vi "16_LinesDecoder.vi"(3 "ENABLED":bool=TRUE, 4 "Integer 0..15  (0)":i32 min=0 max=15) -> (1 "decoded drives":T1)   [LabVIEW 2012]
doc: "Used by Scanner with R and T displays.vi."
panel:
  # "Integer 0..15 to  16 Boolean lines decoder"
  # "0"
  # "15"
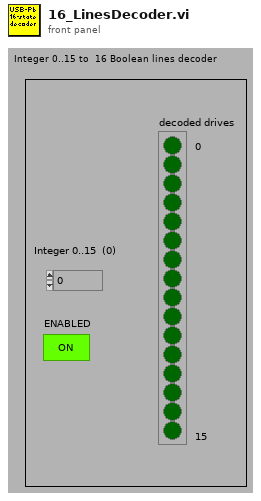
[diagram p1: front panel]
types:
  T1 = cluster{bool, bool, bool, bool, bool, bool, bool, bool, bool, bool, bool, bool, bool, bool, bool, bool}
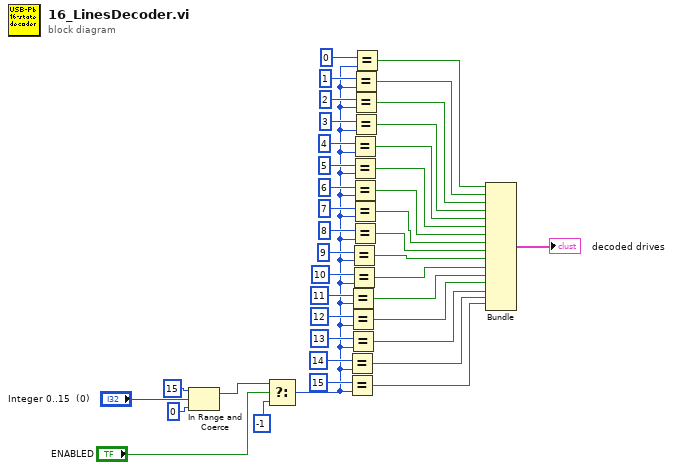
[diagram p0: block diagram]
diagram:
  n1 = In Range and Coerce(upper limit=15, x="Integer 0..15  (0)", lower limit=0) -> (coerced(x)=w3:i32)  [unwired: 1 out]
  n2 = Select(t=w3, s="ENABLED", f=-1) -> (s? t:f=w4:i32)
  n3 = Equal?(x=14, y=w4) -> (x = y?=w23:bool)
  n4 = Equal?(x=15, y=w4) -> (x = y?=w24:bool)
  n5 = Equal?(x=11, y=w4) -> (x = y?=w20:bool)
  n6 = Equal?(x=12, y=w4) -> (x = y?=w21:bool)
  n7 = Equal?(x=13, y=w4) -> (x = y?=w22:bool)
  n8 = Equal?(x=9, y=w4) -> (x = y?=w18:bool)
  n9 = Equal?(x=10, y=w4) -> (x = y?=w19:bool)
  n10 = Equal?(x=4, y=w4) -> (x = y?=w13:bool)
  n11 = Equal?(x=5, y=w4) -> (x = y?=w14:bool)
  n12 = Equal?(x=6, y=w4) -> (x = y?=w15:bool)
  n13 = Equal?(x=7, y=w4) -> (x = y?=w16:bool)
  n14 = Equal?(x=8, y=w4) -> (x = y?=w17:bool)
  n15 = Equal?(x=1, y=w4) -> (x = y?=w10:bool)
  n16 = Equal?(x=2, y=w4) -> (x = y?=w11:bool)
  n17 = Equal?(x=3, y=w4) -> (x = y?=w12:bool)
  n18 = Equal?(x=0, y=w4) -> (x = y?=w9:bool)
  n19 = Bundle(w9, w10, w11, w12, w13, w14, w15, w16, w17, w18, w19, w20, w21, w22, w23, w24) -> (→"decoded drives":T1)  [unwired: 1 in]
